vi "save_calib.vi"(8 "error in (no error)":errorcluster, 9 "name sample":string, 10 "Save Path":path, 11 "Param. Calib":T1) -> (0 "error out":errorcluster)   [LabVIEW 2023]
uses:
  control/param_calibrazione.ctl
  <vilib>/Utility/file.llb/Write Delimited Spreadsheet (string).vi
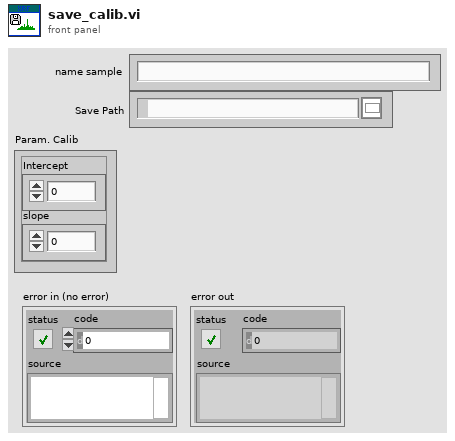
[diagram p1: front panel]
types:
  T1 = typedef "param_calibrazione.ctl" = cluster{"Intercept":dbl, "slope":dbl}
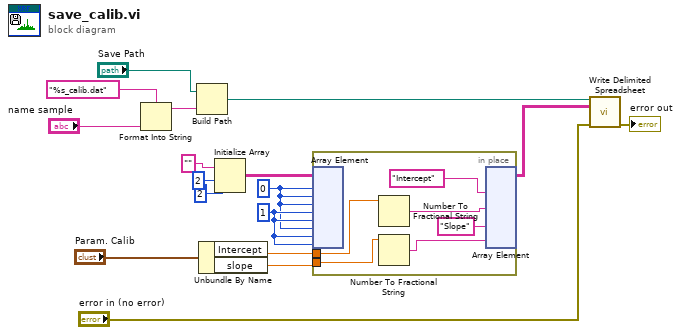
[diagram p0: block diagram]
diagram:
  w14 = 1
  w13 = 0
  n1 = Format Into String(format string="%s_calib.dat", "name sample") -> (resulting string=w6:string)  [unwired: 2 in, 1 out]
  n2 = Build Path(base path="Save Path", name or relative path=w6) -> (appended path=w3:path)
  n3 = Unbundle By Name("Param. Calib") -> ("Intercept"=w11:dbl, "slope"=w10:dbl)
  n4 = Initialize Array("", 2 ("dimension size"), 2 ("dimension size")) -> (w12:string[][])
  n5 = in-place {
    in-place-border: w11 -> [w21]
    in-place-border: w10 -> [w20]
    n6 = in-place-array #1(w12, w13, w13, w13, w14, w14, w13, w14, w14) -> ()  [unwired: 4 out]
    n7 = Number To Fractional String(number=w21) -> (F-format string=w18:string)  [unwired: 3 in]
    n8 = Number To Fractional String(number=w20) -> (F-format string=w19:string)  [unwired: 3 in]
    n9 = in-place-array #1("Intercept", w18, "Slope", w19) -> (w4:string[][])  [unwired: 8 out]
  }
  n10 = call-poly <vilib>:"Write Delimited Spreadsheet.vi"("file path (dialog if empty)"=w3, "2D data"=w4, "error in (no error)"="error in (no error)") -> ("error out"=→"error out":errorcluster)  [unwired: 11 in, 1 out]
